vi "Accel Buffer Check.vi"(11 "00-02-9234 Raw in":dbl[](array[numeric])) -> (2 "size(s)":i32, 3 "00-02-9234 Raw out":dbl[](array[numeric]))   [LabVIEW 2014, in "RT - Analysis.lvlib"]
uses:
  RT - Analysis.lvlib
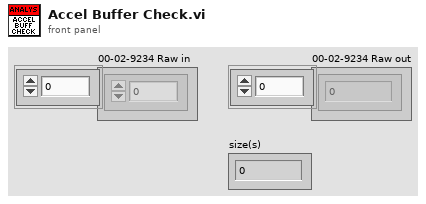
[diagram p1: front panel]
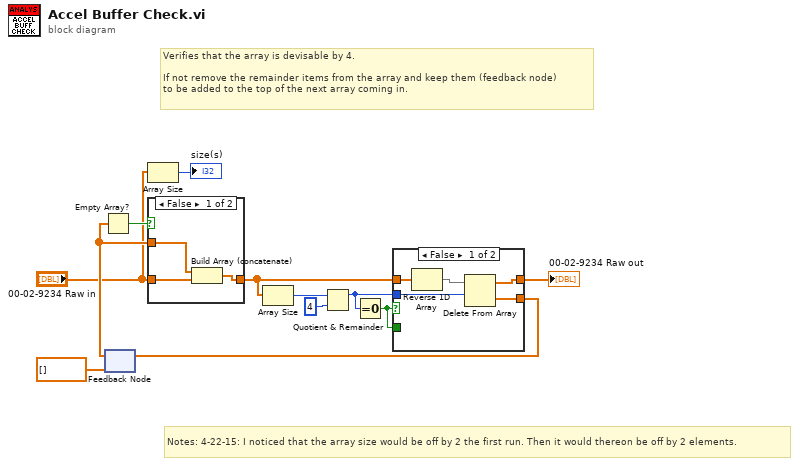
[diagram p0: block diagram]
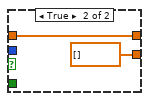
[diagram p3: hidden frame]
diagram:
  # "Notes: 4-22-15: I noticed that the array size would be off by 2 the first run. Then it would thereon be off by 2 elements."
  # "Verifies that the array is devisable by 4. \n\nIf not remove the remainder items from the array and keep them (feedback node)\nto be added to the top of the next array coming in."
  n1 = feedback #1(dbl[] []) -> (w11:dbl[])
  n2 = Empty Array?(array=w11) -> (empty?=w10:bool)
  n3 = Array Size(array="00-02-9234 Raw in") -> (size(s)=→"size(s)":i32)
  n4 = case shown="False" w10 {
    tunnel: "00-02-9234 Raw in" -> [w14 w16]
    tunnel: [w13 w16] -> w6
    tunnel: w11 -> [w15 _]
    frame False {
      n5 = Build Array (concatenate)(w15, w14) -> (w13:dbl[])
    }
    frame True {
    }
  }
  n6 = Array Size(array=w6) -> (size(s)=w2:i32)
  n7 = Quotient & Remainder(x=w2, y=4) -> (x-y*floor(x/y)=w12:i32)  [unwired: 1 out]
  n8 = Equal To 0?(x=w12) -> (x = 0?=w4:bool)
  n9 = case shown="False" w4 {
    tunnel: w6 -> [w21 w23]
    tunnel: [w18 w23] -> w3
    tunnel: w4 -> [_ _]
    tunnel: w12 -> [w19 _]
    tunnel: [w17 dbl[] []] -> w5
    frame False {
      n10 = Reverse 1D Array(array=w21) -> (reversed array=w20:dbl[])
      n11 = Delete From Array(array=w20, length=w19) -> (deleted portion=w17:dbl[], array with subset deleted=w18:dbl[])  [unwired: 1 in]
    }
    frame True {
    }
  }
  "00-02-9234 Raw out" <- w3
  n12 = feedback-in #1(w5) -> ()
